vi "Close.vi"(8 "error in (no error)":errorcluster, 11 "Encoder Ref In":T1) -> (0 "error out":errorcluster)   [LabVIEW 2021, in "Encoder.lvlib"]
doc: "Closes the reference to an encoder channel, disables the counter, and resets the counter value to zero."
uses:
  <vilib>/myRIO/Instrument Drivers/Onboard IO/Encoder/Encoder.lvlib
  <vilib>/myRIO/Instrument Drivers/Onboard IO/Encoder/typedefs/Encoder Reference.ctl
  <vilib>/myRIO/Common/Instrument Driver Framework/Utilities/typedefs/myRIO Generic Hardware Reference.ctl
  <vilib>/myRIO/Common/Instrument Driver Framework/Utilities/typedefs/Hardware Version Enum.ctl
  <vilib>/myRIO/Common/Instrument Driver Framework/Utilities/typedefs/myRIO v1.0 Reference.ctl
  <vilib>/myRIO/Common/Instrument Driver Framework/Utilities/typedefs/Generic FPGA Reference.ctl
  <vilib>/myRIO/Common/Instrument Driver Framework/myRIO v1.0/Encoder/typedefs/Encoder Channels Enum.ctl
  <vilib>/myRIO/Common/Instrument Driver Framework/myRIO v1.0/Encoder/vis/myRIO v1.0 Unreserve Encoder.vi
  <vilib>/myRIO/Common/Instrument Driver Framework/roboRIO v1.0/Encoder/vis/roboRIO v1.0 Unreserve Encoder.vi
  <vilib>/myRIO/Common/Instrument Driver Framework/ELVIS III v1.0/Encoder/vis/ELVIS III v1.0 Unreserve Encoder.vi
  <vilib>/myRIO/Common/Instrument Driver Framework/myRIO v1.0/Encoder/vis/myRIO v1.0 Build MUX Configuration Encoder.vi
  <vilib>/myRIO/Common/Instrument Driver Framework/myRIO v1.0/Resource Manager/vis/myRIO v1.0 Unreserve Channel List.vi
  <vilib>/myRIO/Common/Instrument Driver Framework/roboRIO v1.0/Resource Manager/vis/roboRIO v1.0 Unreserve Channel List.vi
  <vilib>/myRIO/Common/Instrument Driver Framework/roboRIO v1.0/Encoder/vis/roboRIO v1.0 Build MUX Configuration Encoder.vi
  <vilib>/myRIO/Common/Instrument Driver Framework/ELVIS III v1.0/Encoder/vis/ELVIS III v1.0 Build MUX Configuration Encoder.vi
  <vilib>/myRIO/Common/Instrument Driver Framework/myRIO v1.0/Resource Manager/vis/myRIO v1.0 Create Configuration List.vi
  <vilib>/myRIO/Common/Instrument Driver Framework/myRIO v1.0/Resource Manager/vis/myRIO v1.0 Unreserve Channel.vi
  <vilib>/myRIO/Common/Instrument Driver Framework/roboRIO v1.0/Resource Manager/vis/roboRIO v1.0 Unreserve Channel.vi
  <vilib>/myRIO/Common/Instrument Driver Framework/roboRIO v1.0/Resource Manager/vis/roboRIO v1.0 Create Configuration List.vi
  <vilib>/myRIO/Common/Instrument Driver Framework/ELVIS III v1.0/Resource Manager/vis/ELVIS III v1.0 Create Configuration List.vi
  <vilib>/myRIO/Common/Instrument Driver Framework/myRIO v1.0/Resource Manager/vis/myRIO v1.0 Build Mutex Name.vi
  <vilib>/myRIO/Common/Instrument Driver Framework/roboRIO v1.0/Resource Manager/vis/roboRIO v1.0 Build Mutex Name.vi
  <vilib>/myRIO/Common/Instrument Driver Framework/myRIO v1.0/Encoder/vis/myRIO v1.0 Shutdown Encoder.vi
  <vilib>/myRIO/Common/Instrument Driver Framework/myRIO v1.0/Resource Manager/vis/myRIO v1.0 Configure IO.vi
  <vilib>/myRIO/Common/Instrument Driver Framework/Utilities/vis/Configuration Manager.vi
  <vilib>/myRIO/Common/Instrument Driver Framework/Utilities/vis/IO Manager.vi
  <vilib>/myRIO/Common/Instrument Driver Framework/roboRIO v1.0/Encoder/vis/roboRIO v1.0 Shutdown Encoder.vi
  <vilib>/myRIO/Common/Instrument Driver Framework/roboRIO v1.0/Resource Manager/vis/roboRIO v1.0 Configure IO.vi
  <vilib>/myRIO/Common/Instrument Driver Framework/ELVIS III v1.0/Encoder/vis/ELVIS III v1.0 Shutdown Encoder.vi
  <vilib>/myRIO/Common/Instrument Driver Framework/ELVIS III v1.0/Resource Manager/vis/ELVIS III v1.0 Configure IO.vi
  <vilib>/myRIO/Common/Instrument Driver Framework/ELVIS III v1.0/Resource Manager/vis/ELVIS III v1.0 Unreserve Channel List.vi
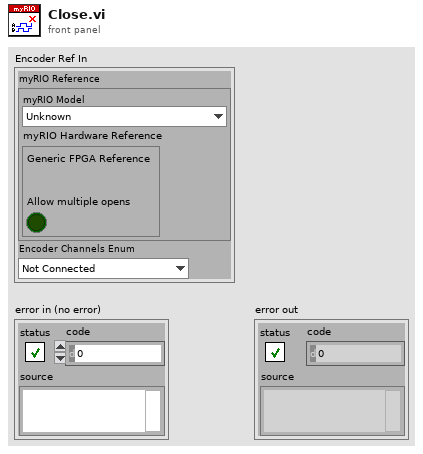
[diagram p1: front panel]
types:
  T1 = typedef "Encoder.lvlib/Encoder Reference.ctl" = cluster{"myRIO Reference":T2, "Encoder Channels Enum":T6}
  T2 = typedef "myRIO Generic Hardware Reference.ctl" = cluster{"myRIO Model":T3, "myRIO Hardware Reference":T4}
  T3 = typedef "Hardware Version Enum.ctl" = enum16{"Unknown", "myRIO-1900", "myRIO-1950", "roboRIO", "NI ELVIS RIO CM", "ELVIS III"}
  T4 = typedef "myRIO v1.0 Reference.ctl" = cluster{"Generic FPGA Reference":T5, "Allow multiple opens":bool}
  T5 = typedef "Generic FPGA Reference.ctl" = refnum<k20>
  T6 = typedef "Encoder Channels Enum.ctl" = enum16{"Not Connected", "C/ENC0", "C/ENC1", "A/ENC", "A/ENC0", "A/ENC1", "A/ENC2", "A/ENC3", "A/ENC4", "A/ENC5", "A/ENC6", "A/ENC7", "A/ENC8", "A/ENC9", "B/ENC", "B/ENC0", "B/ENC1", "B/ENC2", "B/ENC3", "B/ENC4", "B/ENC5", "B/ENC6", "B/ENC7", "B/ENC8", "B/ENC9", "DIO/ENC0", "DIO/ENC1", "DIO/ENC2", "DIO/ENC3", "DIO/ENC4"}
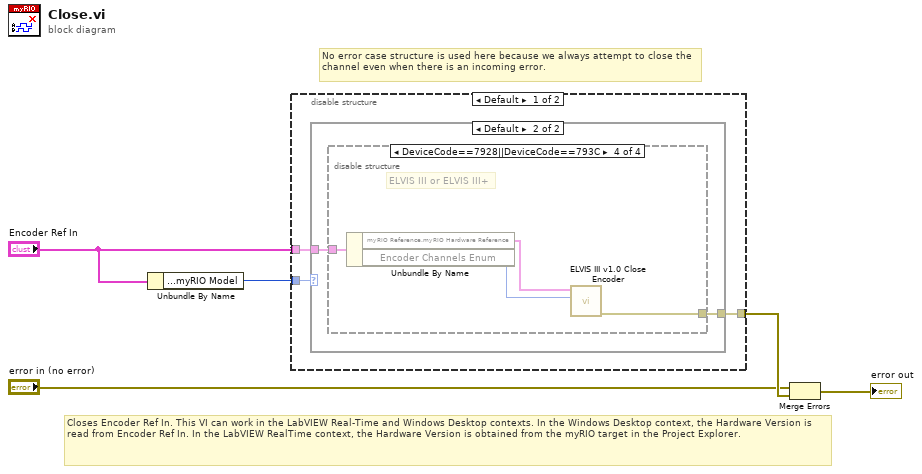
[diagram p0: block diagram]
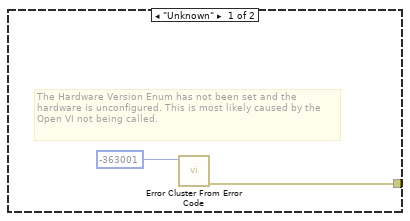
[diagram p2: hidden frame]
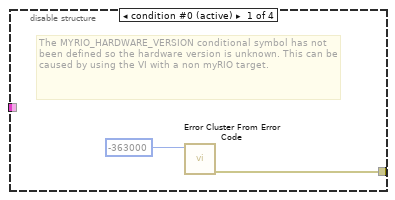
[diagram p3: hidden frame]
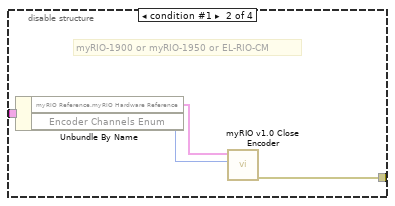
[diagram p4: hidden frame]
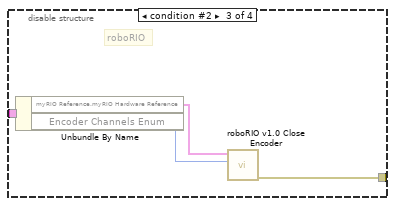
[diagram p5: hidden frame]
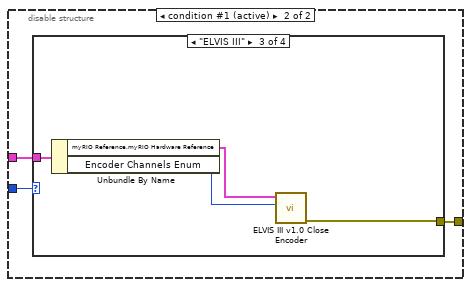
[diagram p6: hidden frame]
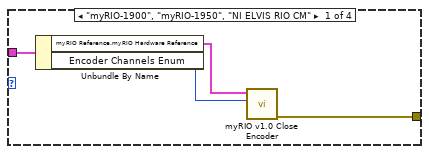
[diagram p7: hidden frame]
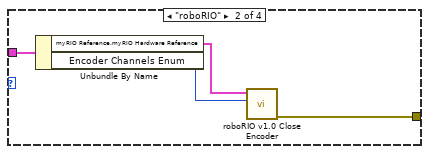
[diagram p8: hidden frame]
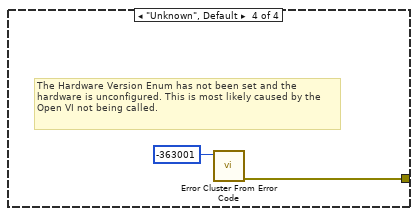
[diagram p9: hidden frame]
diagram:
  # "No error case structure is used here because we always attempt to close the channel even when there is an incoming error."
  # "Closes Encoder Ref In. This VI can work in the LabVIEW Real-Time and Windows Desktop contexts. In the Windows Desktop context, the Hardware Version is read from Encoder Ref In. In the LabVIEW RealTime context, the Hardware Version is obtained from the myRIO target in the Project Explorer."
  n1 = Unbundle By Name("Encoder Ref In") -> ("myRIO Reference.myRIO Model"=w1:T3)
  n2 = disable-structure shown="Default" {
    disable-tunnel: "Encoder Ref In" -> [w8 w28]
    disable-tunnel: [w7 w29] -> w5
    disable-tunnel: w1 -> [w6 w27]
    frame condition #0 {
      n3 = case shown="Default" w6 {
        tunnel: w8 -> [_ w12]
        tunnel: [w9 w11] -> w7
        frame "Unknown" {
          # "The Hardware Version Enum has not been set and the hardware is unconfigured. This is most likely caused by the Open VI not being called."
          n4 = call <vilib>:"Error Cluster From Error Code.vi"("error code (0)"=-363001) -> ("error out"=w9:errorcluster)  [unwired: 8 in]
        }
        frame Default {
          n5 = disable-structure shown="DeviceCode==7928||DeviceCode==793C" {
            disable-tunnel: w12 -> [_ w18 w22 w26]
            disable-tunnel: [w13 w17 w21 w23] -> w11
            frame condition #0 (active) {
              # "The MYRIO_HARDWARE_VERSION conditional symbol has not been defined so the hardware version is unknown. This can be caused by using the VI with a non myRIO target."
              n6 = call <vilib>:"Error Cluster From Error Code.vi"("error code (0)"=-363000) -> ("error out"=w13:errorcluster)  [unwired: 8 in]
            }
            frame condition #1 {
              # "myRIO-1900 or myRIO-1950 or EL-RIO-CM"
              n7 = Unbundle By Name(w18) -> ("myRIO Reference.myRIO Hardware Reference"=w16:T4, "Encoder Channels Enum"=w15:T6)
              n8 = call <vilib>:"myRIO v1.0 Close Encoder.vi"("Encoder Channel"=w15, "myRIO Ref In"=w16) -> ("error out"=w17:errorcluster)  [unwired: 9 in]
            }
            frame condition #2 {
              # "roboRIO"
              n9 = Unbundle By Name(w22) -> ("myRIO Reference.myRIO Hardware Reference"=w20:T4, "Encoder Channels Enum"=w19:T6)
              n10 = call <vilib>:"roboRIO v1.0 Close Encoder.vi"("Encoder Channel"=w19, "myRIO Ref In"=w20) -> ("error out"=w21:errorcluster)  [unwired: 9 in]
            }
            frame condition #3 {
              # "ELVIS III or ELVIS III+"
              n11 = Unbundle By Name(w26) -> ("myRIO Reference.myRIO Hardware Reference"=w25:T4, "Encoder Channels Enum"=w24:T6)
              n12 = call <vilib>:"ELVIS III v1.0 Close Encoder.vi"("Encoder Channel"=w24, "myRIO Ref In"=w25) -> ("error out"=w23:errorcluster)  [unwired: 9 in]
            }
          }
        }
      }
    }
    frame condition #1 (active) {
      n13 = case shown="\"ELVIS III\"" w27 {
        tunnel: w28 -> [w33 w37 w39 _]
        tunnel: [w32 w36 w38 w42] -> w29
        frame "myRIO-1900", "myRIO-1950", "NI ELVIS RIO CM" {
          n14 = Unbundle By Name(w33) -> ("myRIO Reference.myRIO Hardware Reference"=w31:T4, "Encoder Channels Enum"=w30:T6)
          n15 = call <vilib>:"myRIO v1.0 Close Encoder.vi"("Encoder Channel"=w30, "myRIO Ref In"=w31) -> ("error out"=w32:errorcluster)  [unwired: 9 in]
        }
        frame "roboRIO" {
          n16 = Unbundle By Name(w37) -> ("myRIO Reference.myRIO Hardware Reference"=w35:T4, "Encoder Channels Enum"=w34:T6)
          n17 = call <vilib>:"roboRIO v1.0 Close Encoder.vi"("Encoder Channel"=w34, "myRIO Ref In"=w35) -> ("error out"=w36:errorcluster)  [unwired: 9 in]
        }
        frame "ELVIS III" {
          n18 = Unbundle By Name(w39) -> ("myRIO Reference.myRIO Hardware Reference"=w41:T4, "Encoder Channels Enum"=w40:T6)
          n19 = call <vilib>:"ELVIS III v1.0 Close Encoder.vi"("Encoder Channel"=w40, "myRIO Ref In"=w41) -> ("error out"=w38:errorcluster)  [unwired: 9 in]
        }
        frame "Unknown", Default {
          # "The Hardware Version Enum has not been set and the hardware is unconfigured. This is most likely caused by the Open VI not being called."
          n20 = call <vilib>:"Error Cluster From Error Code.vi"("error code (0)"=-363001) -> ("error out"=w42:errorcluster)  [unwired: 8 in]
        }
      }
    }
  }
  n21 = Merge Errors("error in (no error)", w5) -> (→"error out":errorcluster)
